vi "Write Select Report File.vi"(8 "error in (no error)":errorcluster, 10 "Select Report File":path, 11 "Select Report File Dialog in":refnum<class "Select Report File Dialog.lvclass">) -> (0 "error out":errorcluster, 3 "Select Report File Dialog out":refnum<class "Select Report File Dialog.lvclass">)   [LabVIEW 2014, in "Select Report File Dialog.lvlib" / "Select Report File Dialog.lvclass"]
uses:
  Select Report File Dialog.lvclass
  Select Report File Dialog.lvclass/Select Report File Dialog.ctl
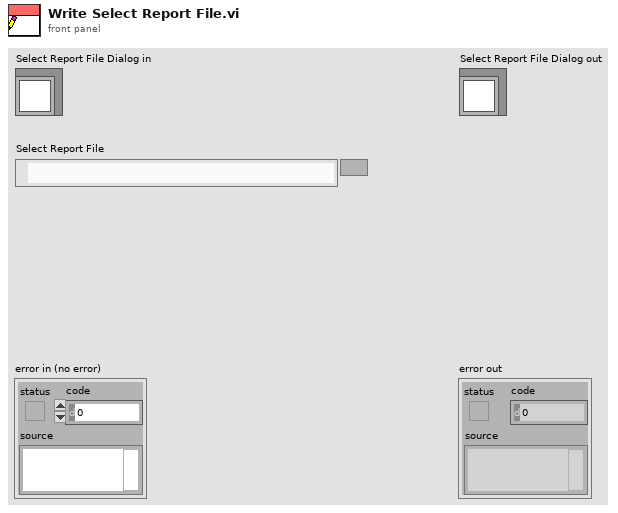
[diagram p1: front panel]
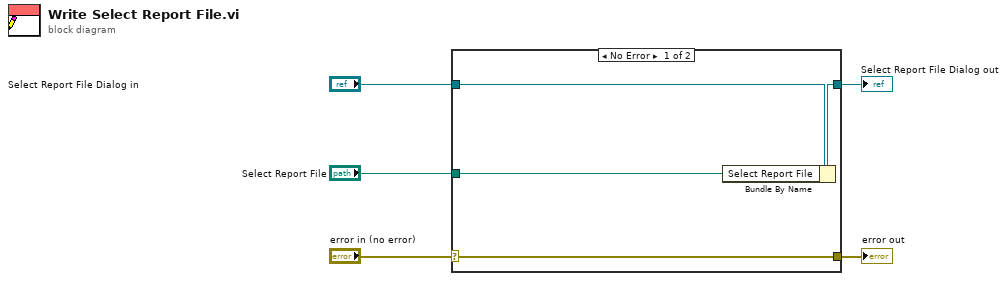
[diagram p0: block diagram]
diagram:
  n1 = case shown="No Error" "error in (no error)" {
    selector: "error in (no error)" -> [w9 w10]
    tunnel: [w9 w10] -> w4
    tunnel: [w7 w11] -> w2
    tunnel: "Select Report File Dialog in" -> [w8 w11]
    tunnel: "Select Report File" -> [w6 _]
    frame No Error {
      n2 = Bundle By Name(cluster=w8, "Select Report File"=w6) -> (w7:refnum<class "Select Report File Dialog.lvclass">)
    }
    frame Error {
    }
  }
  "error out" <- w4
  "Select Report File Dialog out" <- w2
